vi "get-config-daemon.vi"() -> ()   [LabVIEW 2021]
uses:
  daemon-config.ctl
panel:
  out "value":T1={"resource-type"="battery", "agent-id"=12, "GA-ip"="192.168.1.1", "GA-port"=52020, "RA-ip"="127.0.0.1", "RA-port"=52001, "listenport-RA-side"=52011, "listenport-GA-side"=52021, "local-ip"="192.168.1.12", "long-term"=FALSE}
  out "text":string
  in  "path":path
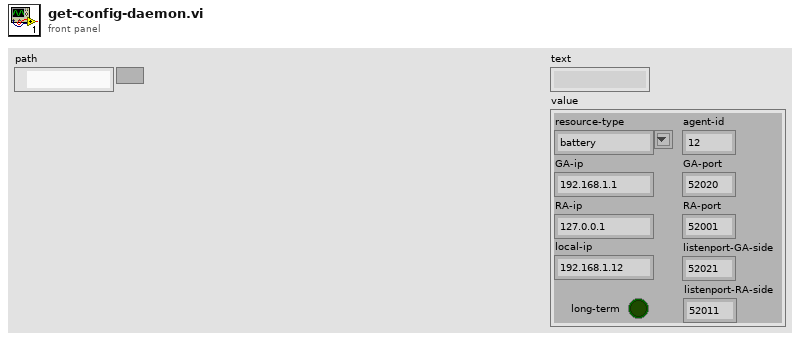
[diagram p1: front panel]
types:
  T1 = typedef "daemon-config.ctl" = cluster{"resource-type":string, "agent-id":u16, "GA-ip":string, "GA-port":u16, "RA-ip":string, "RA-port":u16, "listenport-RA-side":u16, "listenport-GA-side":u16, "local-ip":string, "long-term":bool}
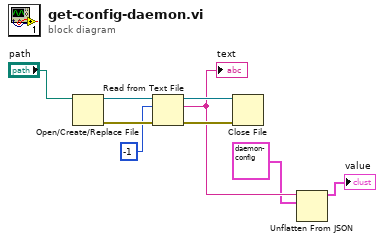
[diagram p0: block diagram]
diagram:
  n1 = Open/Create/Replace File(file path (use dialog)="path") -> (refnum out=w8:refnum<file>, error out=w7:errorcluster)  [unwired: 5 in, 1 out]
  n2 = Read from Text File(file (use dialog)=w8, count=-1, error in=w7) -> (refnum out=w5:refnum<file>, text=w3:string, error out=w4:errorcluster)  [unwired: 1 in, 1 out]
  "text" <- w3
  n3 = Close File(refnum=w5, error in=w4) -> ()  [unwired: 2 out]
  n4 = Unflatten From JSON(JSON string=w3, type and defaults=T1 {"resource-type"="battery", "agent-id"=12, "GA-ip"="192.168.1.1", "GA-port"=52020, "RA-ip"="127.0.0.1", "RA-port"=52001, "listenport-RA-side"=52011, "listenport-GA-side"=52021, "local-ip"="192.168.1.12", "long-term"=FALSE} ("daemon-config")) -> (value=→"value":T1)  [unwired: 5 in, 1 out]
